vi "ReactorMathscript.vi"(0 "T":dbl[][](array[numeric]), 2 "CurCycle":i32, 5 "TPos":i32, 7 "Run":bool) -> (9 "PrePurge":dbl, 11 "PreDosePump":dbl, 13 "StopRun":bool, 14 "TBrk":i32[](array[numeric]), 15 "Purge":dbl, 17 "Holds":dbl, 19 "Dose":dbl, 20 "TCyc":dbl, 21 "CurCycle 2":i32, 22 "TPos 2":i32, 23 "TLeftStr":string, 24 "Case":i32, 25 "Valve":i32, 26 "PreN2":dbl, 27 "PrePump":dbl)   [LabVIEW 2021]
panel:
  out "error out":errorcluster
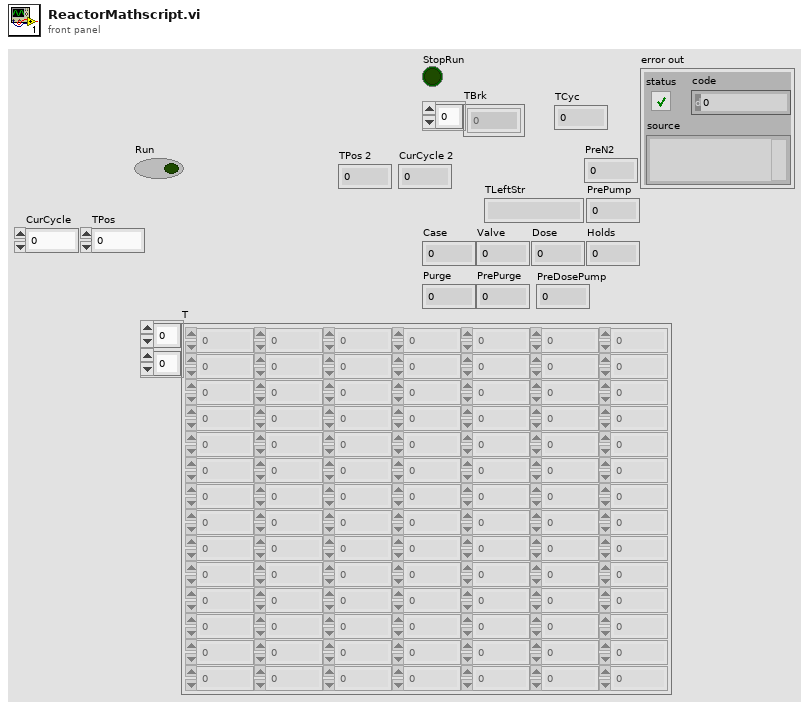
[diagram p1: front panel]
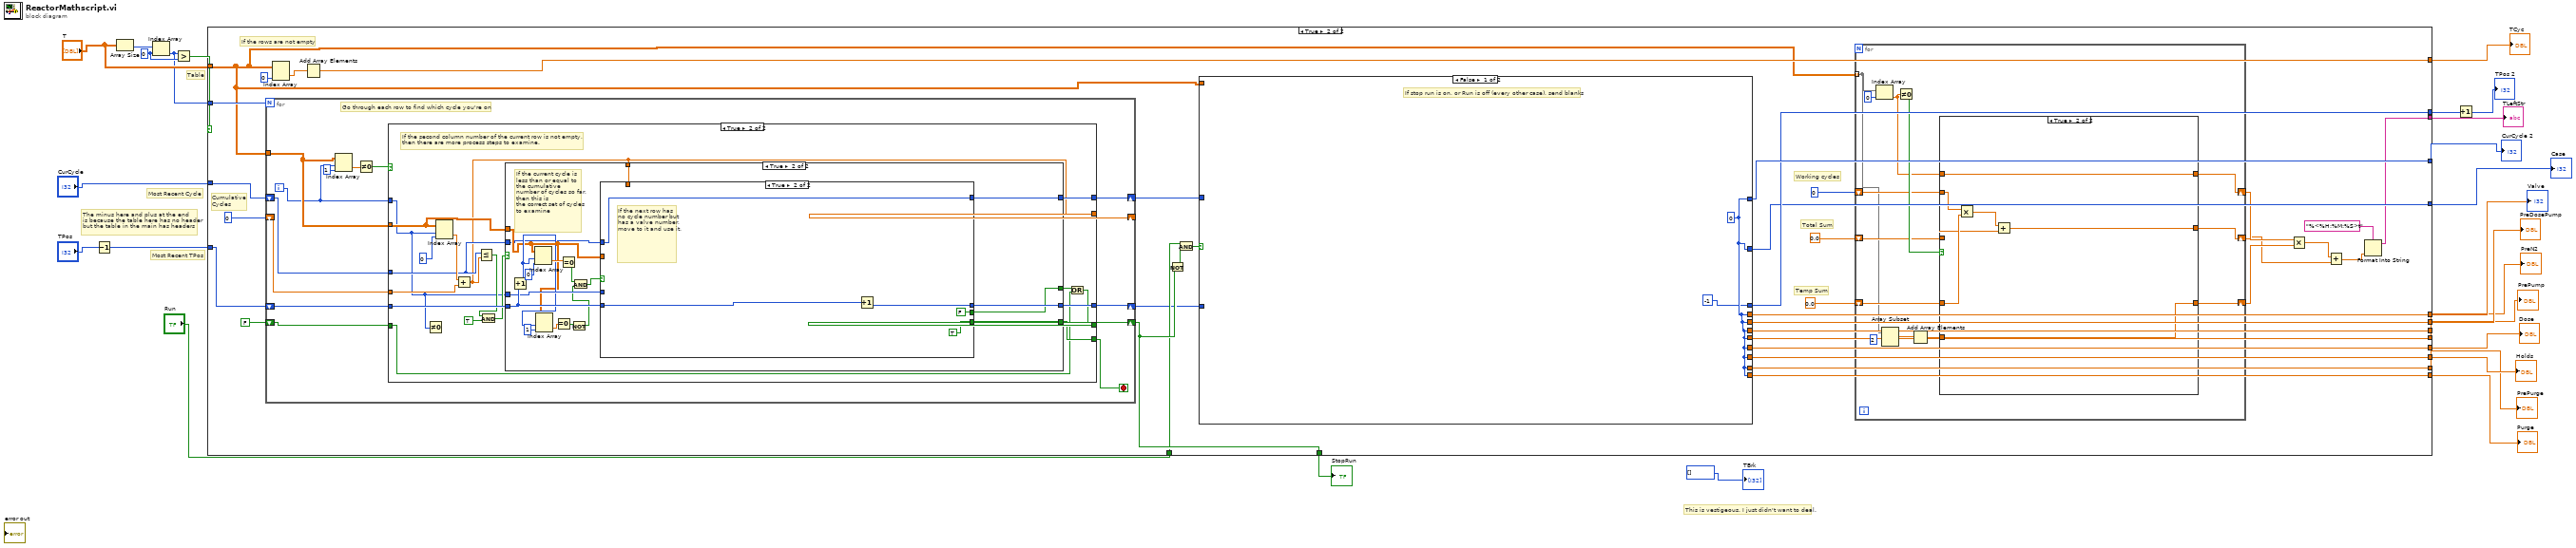
[diagram p0: block diagram]
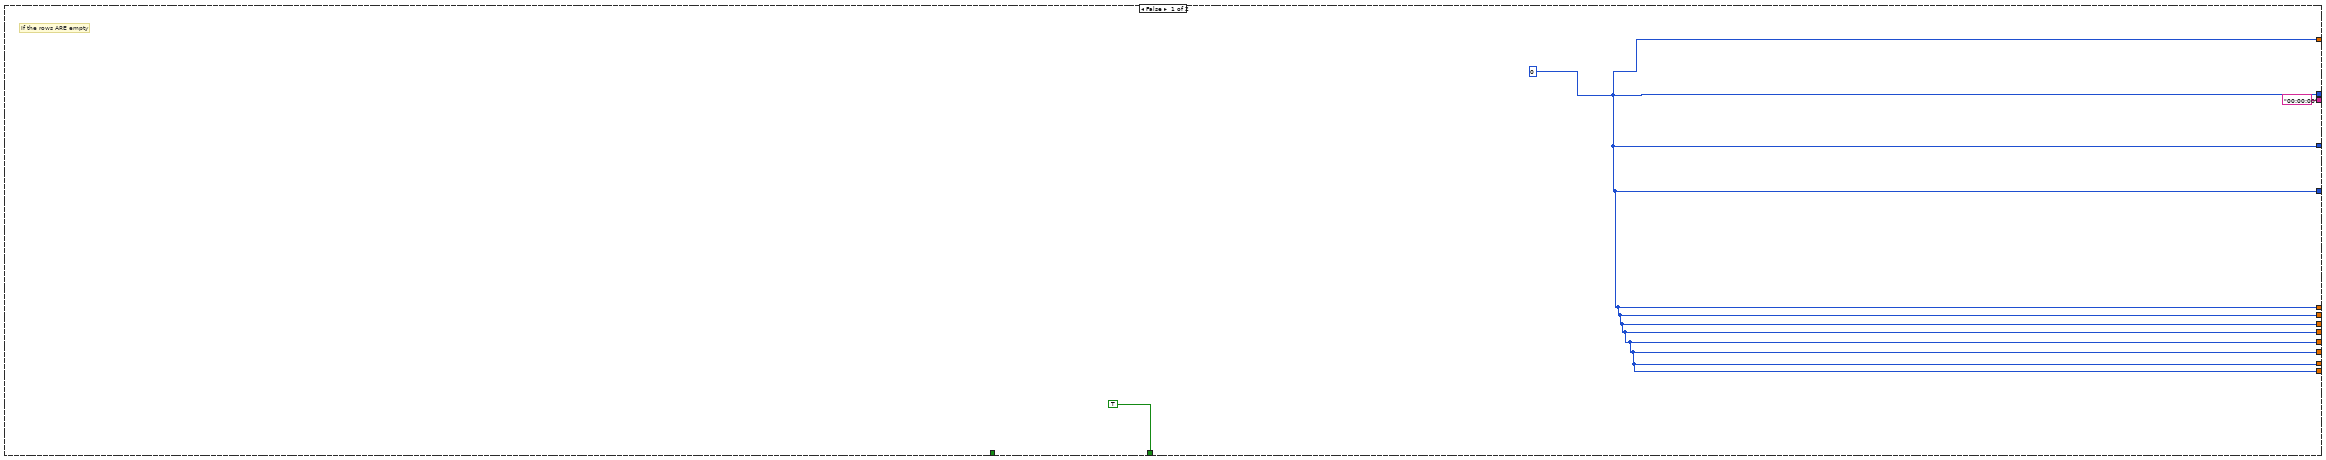
[diagram p2: hidden frame]
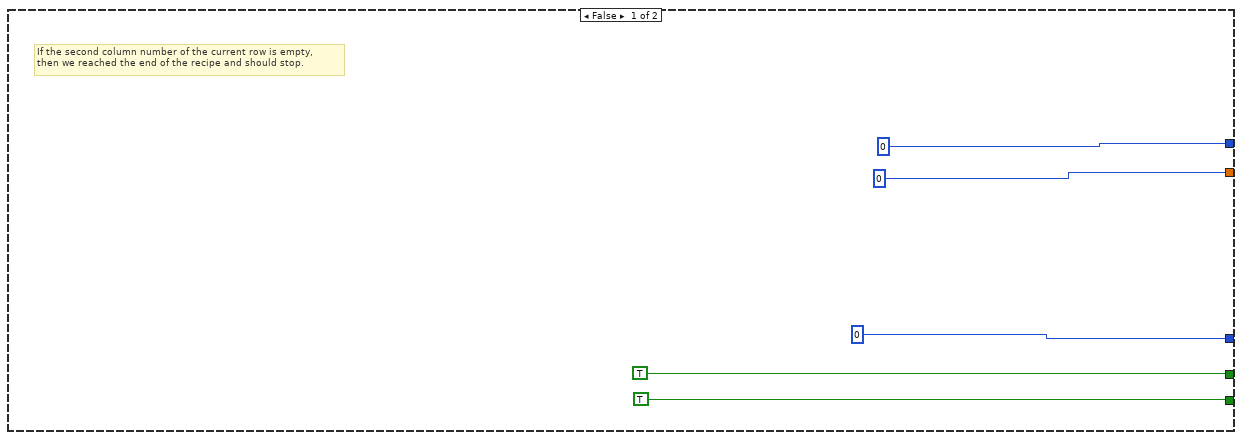
[diagram p3: hidden frame]
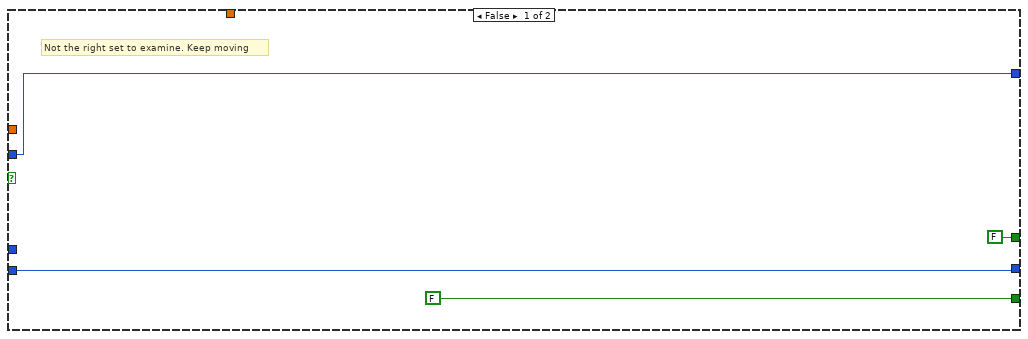
[diagram p4: hidden frame]
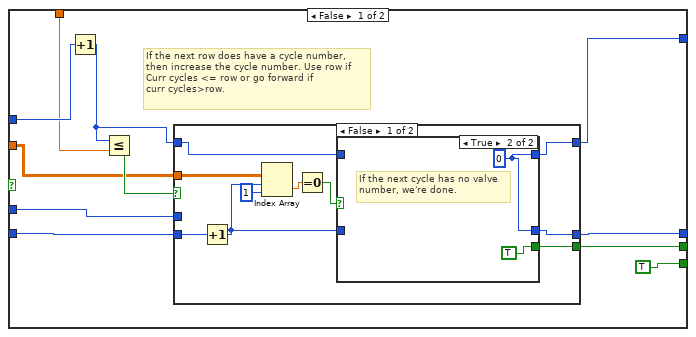
[diagram p5: hidden frame]
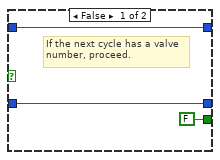
[diagram p6: hidden frame]
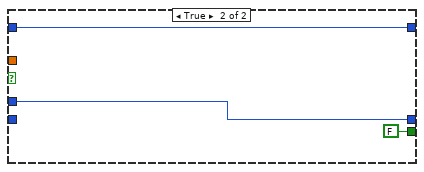
[diagram p7: hidden frame]
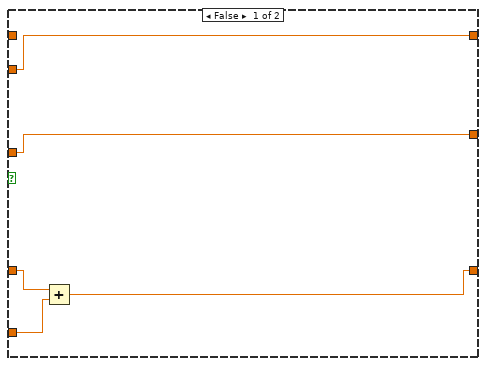
[diagram p8: hidden frame]
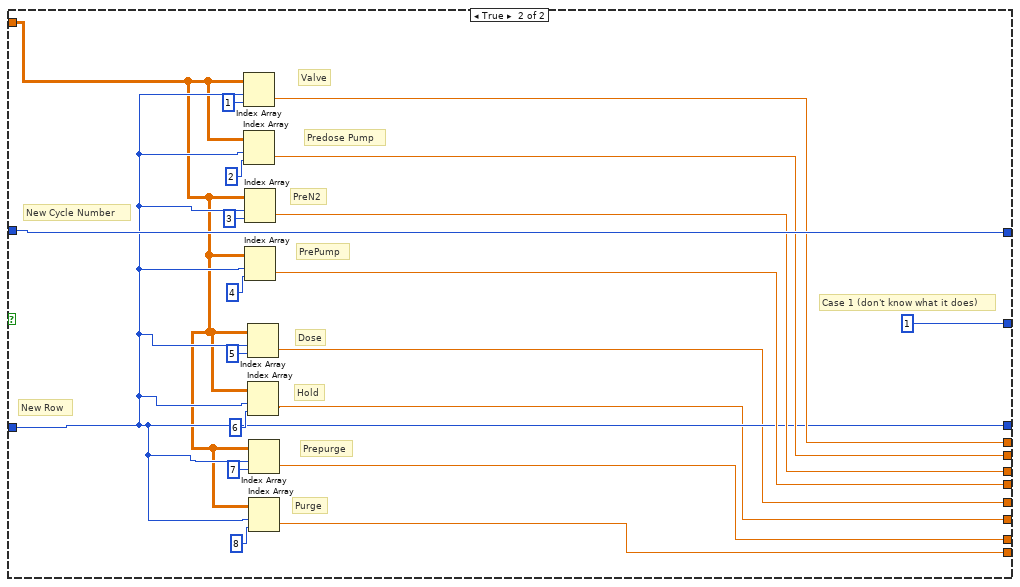
[diagram p9: hidden frame]
diagram:
  w24 = 0 ("index")
  # "The minus here and plus at the end\nis because the table here has no header\nbut the table in the main has headers"
  # "This is vestigeous. I just didn't want to deal."
  # "Most Recent TPos"
  # "Table"
  # "Most Recent Cycle"
  n1 = Decrement(x="TPos") -> (x-1=w1:i32)
  n2 = Array Size(array="T") -> (size(s)=w25:i32[])
  n3 = Index Array(array=w25, index=w24) -> (element=w19:i32)
  n4 = Greater?(x=w19, y=w24) -> (0:w23:bool)
  n5 = case shown="True" w23 {
    tunnel: [w26 w62] -> w22
    tunnel: "T" -> [_ w39]
    tunnel: "CurCycle" -> [_ w59]
    tunnel: w19 -> [_ w61]
    tunnel: w1 -> [_ w58]
    tunnel: [TRUE w55] -> w17
    tunnel: "Run" -> [_ w53]
    tunnel: [w26 w51] -> w15
    tunnel: [w26 w49] -> w14
    tunnel: [w26 w48] -> w13
    tunnel: [w26 w47] -> w12
    tunnel: [w26 w46] -> w11
    tunnel: [w26 w45] -> w10
    tunnel: [w26 w44] -> w9
    tunnel: [w26 w43] -> w8
    tunnel: [w26 w42] -> w7
    tunnel: [w26 w41] -> w6
    tunnel: [w26 w40] -> w5
    tunnel: ["00:00:00" w29] -> w3
    frame False {
      w26 = 0
      # "If the rows ARE empty"
    }
    frame True {
      # "Working cycles"
      # "Total Sum"
      # "Temp Sum"
      # "Cumulative\nCycles"
      # "If the rows are not empty"
      n6 = for {
        N: w61 -> [_]
        tunnel: w39 -> [w75]
        shift-right: [w76] -> _
        shift-left: 0 -> [w78]
        shift-right: [w70] -> w55
        shift-left: FALSE -> [w69]
        shift-right: [w68] -> w50
        shift-left: w58 -> [w71]
        shift-right: [w67] -> w52
        shift-left: w59 -> [w77]
        i -> [w66]
        stop <- w72 stop-if-true
        # "Go through each row to find which cycle you're on"
        n7 = Index Array(array=w75, index (row)=w66, index (col)=1 ("disabled index (col)")) -> (element=w73:dbl)
        n8 = Not Equal To 0?(x=w73) -> (x != 0?=w65:bool)
        n9 = case shown="True" w65 {
          tunnel: w75 -> [_ w97]
          tunnel: w66 -> [_ w89]
          tunnel: w78 -> [_ w98]
          tunnel: w77 -> [_ w92]
          tunnel: [0 w88] -> w76
          tunnel: [TRUE w95] -> w72
          tunnel: w71 -> [_ w96]
          tunnel: [TRUE w85] -> w70
          tunnel: w69 -> [_ w86]
          tunnel: [0 w94] -> w68
          tunnel: [0 w93] -> w67
          frame False {
            # "If the second column number of the current row is empty,\nthen we reached the end of the recipe and should stop."
          }
          frame True {
            # "If the second column number of the current row is not empty,\nthen there are more process steps to examine."
            n10 = Not Equal To 0?(x=w89) -> ()  [unwired: 1 out]
            n11 = Index Array(array=w97, index (row)=w89, index (col)=0 ("disabled index (col)")) -> (element=w99:dbl)
            n12 = Add(x=w99, y=w98) -> (x+y=w88:dbl)
            n13 = Less Or Equal?(x=w92, y=w88) -> (x <= y?=w91:bool)
            n14 = And(x=w91, y=TRUE) -> (x .and. y?=w90:bool)
            n15 = case shown="True" w90 {
              tunnel: w97 -> [_ w115]
              tunnel: w96 -> [w103 w120]
              tunnel: [FALSE w108] -> w95
              tunnel: [w103 w119] -> w94
              tunnel: w92 -> [w102 w107]
              tunnel: [w102 w118] -> w93
              tunnel: w89 -> [_ w117]
              tunnel: w88 -> [_ w106]
              tunnel: [FALSE w105] -> w84
              frame False {
                # "Not the right set to examine. Keep moving"
              }
              frame True {
                # "If the current cycle is\nless than or equal to the cumulative\nnumber of cycles so far, then this is\nthe correct set of cycles to examine"
                n16 = Increment(x=w120) -> (x+1=w116:i32)
                n17 = Index Array(array=w115, index (row)=w116, index (col)=0 ("disabled index (col)")) -> (element=w121:dbl)
                n18 = Index Array(array=w115, index (row)=w116, index (col)=1 ("disabled index (col)")) -> (element=w113:dbl)
                n19 = Equal To 0?(x=w113) -> (x = 0?=w112:bool)
                n20 = Equal To 0?(x=w121) -> (x = 0?=w111:bool)
                n21 = Not(x=w112) -> (.not. x?=w110:bool)
                n22 = And(x=w111, y=w110) -> (x .and. y?=w109:bool)
                n23 = case shown="True" w109 {
                  tunnel: w120 -> [w129 w155]
                  tunnel: [w130 w154] -> w119
                  tunnel: w107 -> [w133 w156]
                  tunnel: [w125 w156] -> w118
                  tunnel: w117 -> [w131 _]
                  tunnel: w115 -> [w124 _]
                  tunnel: [TRUE TRUE] -> w108
                  tunnel: w106 -> [w128 _]
                  tunnel: [w123 FALSE] -> w105
                  frame False {
                    # "If the next row does have a cycle number,\nthen increase the cycle number. Use row if\nCurr cycles <= row or go forward if\ncurr cycles>row."
                    n24 = Increment(x=w133) -> (x+1=w126:i32)
                    n25 = Less Or Equal?(x=w126, y=w128) -> (x <= y?=w132:bool)
                    n26 = case shown="False" w132 {
                      tunnel: w131 -> [_ w151]
                      tunnel: [w135 w151] -> w130
                      tunnel: w129 -> [w143 _]
                      tunnel: w126 -> [w138 w150]
                      tunnel: [w137 w150] -> w125
                      tunnel: w124 -> [w140 _]
                      tunnel: [w134 FALSE] -> w123
                      frame False {
                        n27 = Increment(x=w143) -> (x+1=w136:i32)
                        n28 = Index Array(array=w140, index (row)=w136, index (col)=1 ("disabled index (col)")) -> (element=w142:dbl)
                        n29 = Equal To 0?(x=w142) -> (x = 0?=w139:bool)
                        n30 = case shown="True" w139 {
                          tunnel: w138 -> [w146 _]
                          tunnel: [w146 w148] -> w137
                          tunnel: w136 -> [w145 _]
                          tunnel: [w145 w148] -> w135
                          tunnel: [FALSE TRUE] -> w134
                          frame False {
                            # "If the next cycle has a valve\nnumber, proceed."
                          }
                          frame True {
                            w148 = 0
                            # "If the next cycle has no valve\nnumber, we're done."
                          }
                        }
                      }
                      frame True {
                      }
                    }
                  }
                  frame True {
                    # "If the next row has no cycle number but has a valve number, move to it and use it."
                    n31 = Increment(x=w155) -> (x+1=w154:i32)
                  }
                }
              }
            }
            n32 = Or(x=w84, y=w86) -> (x .or. y?=w85:bool)
          }
        }
      }
      n33 = Index Array(array=w39, index (col)=0 ("disabled index (col)")) -> (element=w63:dbl[])  [unwired: 1 in]
      n34 = Add Array Elements(numeric array=w63) -> (sum=w62:dbl)
      n35 = Not(x=w55) -> (.not. x?=w54:bool)
      n36 = And(x=w53, y=w54) -> (x .and. y?=w56:bool)
      n37 = case shown="False" w56 {
        tunnel: w52 -> [_ w203]
        tunnel: [w183 w203] -> w51
        tunnel: w50 -> [_ w189]
        tunnel: [-1 w189] -> w49
        tunnel: [w183 1] -> w48
        tunnel: w39 -> [_ w188]
        tunnel: [w183 w200] -> w47
        tunnel: [w183 w198] -> w46
        tunnel: [w183 w195] -> w45
        tunnel: [w183 w194] -> w44
        tunnel: [w183 w187] -> w43
        tunnel: [w183 w186] -> w42
        tunnel: [w183 w185] -> w41
        tunnel: [w183 w184] -> w40
        frame False {
          w183 = 0
          # "If stop run is on, or Run is off (every other case), send blanks"
        }
        frame True {
          # "Prepurge"
          # "Purge"
          # "Hold"
          # "Dose"
          # "PrePump"
          # "PreN2"
          # "Predose Pump"
          # "Valve"
          # "Case 1 (don't know what it does)"
          # "New Row"
          # "New Cycle Number"
          n38 = Index Array(array=w188, index (row)=w189, index (col)=1 ("disabled index (col)")) -> (element=w200:dbl)
          n39 = Index Array(array=w188, index (row)=w189, index (col)=2 ("disabled index (col)")) -> (element=w198:dbl)
          n40 = Index Array(array=w188, index (row)=w189, index (col)=3 ("disabled index (col)")) -> (element=w195:dbl)
          n41 = Index Array(array=w188, index (row)=w189, index (col)=4 ("disabled index (col)")) -> (element=w194:dbl)
          n42 = Index Array(array=w188, index (row)=w189, index (col)=5 ("disabled index (col)")) -> (element=w187:dbl)
          n43 = Index Array(array=w188, index (row)=w189, index (col)=6 ("disabled index (col)")) -> (element=w186:dbl)
          n44 = Index Array(array=w188, index (row)=w189, index (col)=7 ("disabled index (col)")) -> (element=w185:dbl)
          n45 = Index Array(array=w188, index (row)=w189, index (col)=8 ("disabled index (col)")) -> (element=w184:dbl)
        }
      }
      n46 = for {
        tunnel: w39 -> [w161] mode=indexing
        shift-right: [w163] -> w34
        shift-left: 0 -> [w166]
        shift-right: [w164] -> w32
        shift-left: 0.0 -> [w167]
        shift-right: [w158] -> w33
        shift-left: 0.0 -> [w165]
        n47 = Index Array(array=w161, index=0) -> (element=w162:dbl)
        n48 = Array Subset(array=w161, index=2) -> (w159:dbl[])  [unwired: 1 in]
        n49 = Not Equal To 0?(x=w162) -> (x != 0?=w168:bool)
        n50 = Add Array Elements(numeric array=w159) -> (sum=w157:dbl)
        n51 = case shown="True" w168 {
          tunnel: w167 -> [w171 w178]
          tunnel: w166 -> [w170 w181]
          tunnel: w165 -> [w174 w180]
          tunnel: [w171 w177] -> w164
          tunnel: [w170 w176] -> w163
          tunnel: w162 -> [_ w176]
          tunnel: [w172 w175] -> w158
          tunnel: w157 -> [w173 w175]
          frame False {
            n52 = Add(x=w174, y=w173) -> (x+y=w172:dbl)
          }
          frame True {
            n53 = Multiply(x=w181, y=w180) -> (x*y=w179:dbl)
            n54 = Add(x=w179, y=w178) -> (x+y=w177:dbl)
          }
        }
      }
      n55 = Multiply(x=w34, y=w33) -> (x*y=w35:dbl)
      n56 = Add(x=w35, y=w32) -> (x+y=w31:dbl)
      n57 = Format Into String(format string="%<%H:%M:%S>t", w31) -> (resulting string=w29:string)  [unwired: 2 in, 1 out]
    }
  }
  "TCyc" <- w22
  "CurCycle 2" <- w15
  "TLeftStr" <- w3
  "Case" <- w13
  "Valve" <- w12
  "PreN2" <- w10
  "PrePump" <- w9
  "Dose" <- w8
  "Holds" <- w7
  "Purge" <- w5
  "StopRun" <- w17
  "PreDosePump" <- w11
  "PrePurge" <- w6
  n58 = Increment(x=w14) -> (x+1=→"TPos 2":i32)
  "TBrk" <- i32[] []
